vi "UDP Named Service - PS Server.vi"() -> ()   [LabVIEW 2025]
doc: "Creates a named service and listens on the first available port. When a client connects to the service, it sends a response string to the client.\nAuthor: Scott Hannahs <sth@magnet.fsu.edu>\n\nThis software is licensed for use under the “MIT License\"\nCopyright (c) 2025 Scott Hannahs, sth@sth@magnet.sthnet.net\n\nPermission is hereby granted, free of charge, to any person obtaining a copy of this software and associated documentation files (the \"Software\"), to deal in the Software without restriction, including without limitation the rights to use, copy, modify, merge, publish, distribute, sublicense, and/or sell copies of the Software, and to permit persons to whom the Software is furnished to do so, subject to the following conditions: The above copyright notice and this permission notice shall be included in all copies or substantial portions of the Software.\n\nTHE SOFTWARE IS PROVIDED \"AS IS\", WITHOUT WARRANTY OF ANY KIND, EXPRESS OR IMPLIED, INCLUDING BUT NOT LIMITED TO THE WARRANTIES OF MERCHANTABILITY, FITNESS FOR A PARTICULAR PURPOSE AND NONINFRINGEMENT. IN NO EVENT SHALL THE AUTHORS OR COPYRIGHT HOLDERS BE LIABLE FOR ANY CLAIM, DAMAGES OR OTHER LIABILITY, WHETHER IN AN ACTION OF CONTRACT, TORT OR OTHERWISE, ARISING FROM, OUT OF OR IN CONNECTION WITH THE SOFTWARE OR THE USE OR OTHER DEALINGS IN THE SOFTWARE."
uses:
  <vilib>/Utility/error.llb/Trim Whitespace One-Sided.vi
panel:
  out "Port":u16
  out "String":string
  in  "Stop":bool
  # "Overview: Demonstrates the use of the UDP functions to initialize a named UDP service that can send data to a client VI.\nInstructions:\n1. Run the VI.\n2. Open UDP Named Service - Client.vi and follow the instructions on its front panel.\n3. Click Stop to stop the VI."
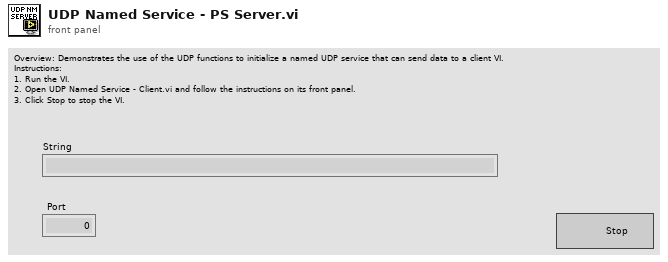
[diagram p1: front panel]
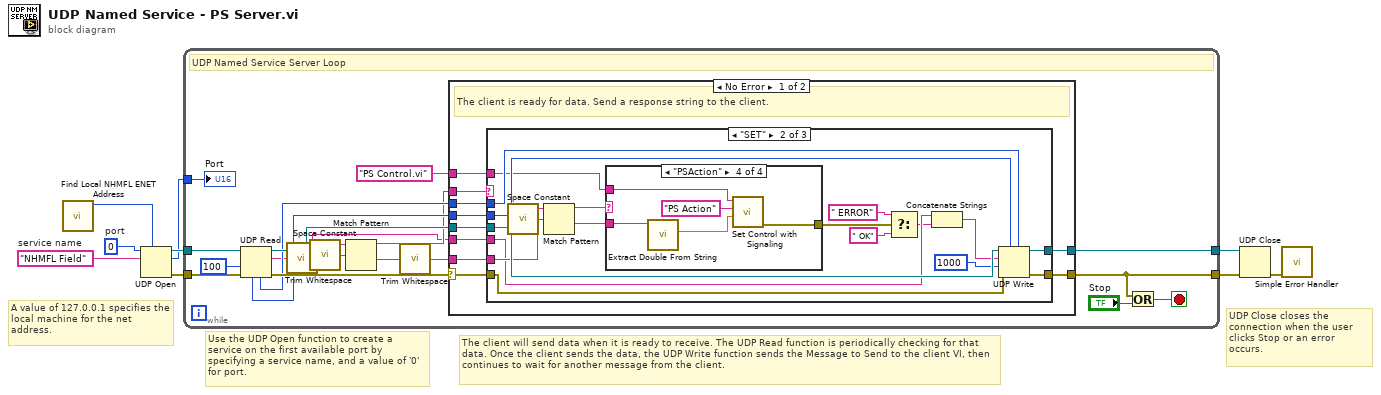
[diagram p0: block diagram]
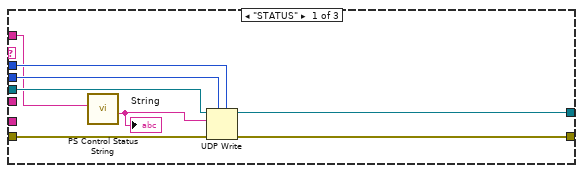
[diagram p2: hidden frame]
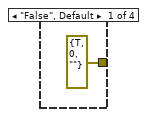
[diagram p3: hidden frame]
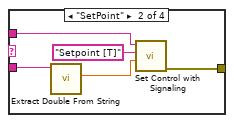
[diagram p4: hidden frame]
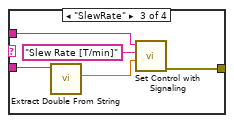
[diagram p5: hidden frame]
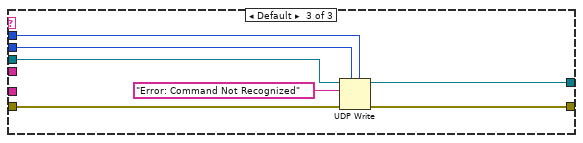
[diagram p6: hidden frame]
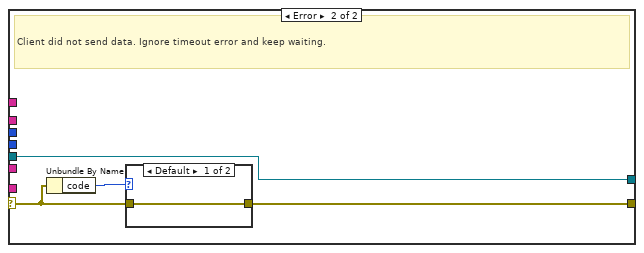
[diagram p7: hidden frame]
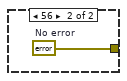
[diagram p8: hidden frame]
diagram:
  w2 = u16 0  # port
  w9 = "NHMFL Field"  # service name
  # "UDP Close closes the connection when the user clicks Stop or an error occurs."
  # "A value of 127.0.0.1 specifies the local machine for the net address."
  # "The client will send data when it is ready to receive. The UDP Read function is periodically checking for that data. Once the client sends the data, the UDP Write function sends the Message to Send to the client VI, then continues to wait for another message from the client."
  # "Use the UDP Open function to create a service on the first available port by specifying a service name, and a value of '0' for port."
  n1 = call "Find Local NHMFL ENET Address.vi"() -> ("Ethernet Address"=w1:u32)  [unwired: 9 in, 2 out]
  n2 = UDP Open(7:w1, 10:w9, 11:w2) -> (port=w8:refnum<k16>, 0:w7:errorcluster, 2:w4:u16)  [unwired: 2 in]
  n3 = while {
    tunnel: [w19] -> w5
    tunnel: w8 -> [w28]
    tunnel: w7 -> [w24]
    tunnel: [w25] -> w6
    tunnel: w4 -> [w22]
    stop <- w21 stop-if-true
    # "UDP Named Service Server Loop"
    n4 = UDP Read(connection ID=w28, timeout ms (25000)=100, 8:w24) -> (data out=w12:string, error out=w27:errorcluster, 3:w26:refnum<k16>, 4:w23:u16, 6:w17:u32)  [unwired: 1 in]
    n5 = call <vilib>:"Trim Whitespace.vi"("string"=w12) -> ("trimmed string"=w10:string)  [unwired: 1 in]
    n6 = call <vilib>:"Space Constant.vi"() -> ("String"=w13:string)
    n7 = Match Pattern(string=w10, regular expression=w13) -> (before substring=w16:string, after substring=w15:string)  [unwired: 1 in, 2 out]
    n8 = call <vilib>:"Trim Whitespace.vi"("string"=w15) -> ("trimmed string"=w14:string)  [unwired: 1 in]
    n9 = case shown="No Error" w27 {
      selector: w27 -> [w38 w90]
      tunnel: w26 -> [w35 w91]
      tunnel: [w37 w88] -> w19
      tunnel: [w36 w91] -> w25
      tunnel: w17 -> [w33 _]
      tunnel: w23 -> [w34 _]
      tunnel: w16 -> [w32 _]
      tunnel: w14 -> [w31 _]
      tunnel: w10 -> [w30 _]
      tunnel: "PS Control.vi" -> [w29 _]
      frame No Error {
        # "The client is ready for data. Send a response string to the client."
        n10 = case shown="\"SET\"" w32 {
          tunnel: w38 -> [w46 w64 w87]
          tunnel: [w45 w63 w86] -> w37
          tunnel: [w44 w62 w85] -> w36
          tunnel: w35 -> [w43 w61 w84]
          tunnel: w34 -> [w42 w60 w83]
          tunnel: w33 -> [w41 w59 w82]
          tunnel: w31 -> [_ w58 _]
          tunnel: w30 -> [_ w54 _]
          tunnel: w29 -> [w39 w47 _]
          frame "STATUS" {
            n11 = call "PS Control Status String.vi"("VI Name"=w39) -> ("Status String"=w40:string)  [unwired: 9 in, 1 out]
            "String" <- w40
            n12 = UDP Write(address=w41, port or service name=w42, connection ID=w43, data in=w40, 8:w46) -> (error out=w45:errorcluster, 3:w44:refnum<k16>)  [unwired: 1 in]
          }
          frame "SET" {
            n13 = call <vilib>:"Space Constant.vi"() -> ("String"=w57:string)
            n14 = Match Pattern(string=w58, regular expression=w57) -> (before substring=w56:string, after substring=w55:string)  [unwired: 1 in, 2 out]
            n15 = case shown="\"PSAction\"" w56 {
              tunnel: w55 -> [_ w67 w72 w77]
              tunnel: w47 -> [_ w69 w74 w79]
              tunnel: [errorcluster {"status"=TRUE, "code"=0, "source"=""} ("error out") w66 w71 w76] -> w53
              frame "False", Default {
              }
              frame "SetPoint" {
                n16 = call "Extract Double From String.vi"("string"=w67) -> ("floating pt. number"=w68:dbl)  [unwired: 3 in, 3 out]
                n17 = call "Set Control with Signaling.vi"("Value"=w68, "Control Name"="Setpoint [T]", "VI Name"=w69) -> ("error out"=w66:errorcluster)  [unwired: 8 in]
              }
              frame "SlewRate" {
                n18 = call "Extract Double From String.vi"("string"=w72) -> ("floating pt. number"=w73:dbl)  [unwired: 3 in, 3 out]
                n19 = call "Set Control with Signaling.vi"("Value"=w73, "Control Name"="Slew Rate [T/min]", "VI Name"=w74) -> ("error out"=w71:errorcluster)  [unwired: 8 in]
              }
              frame "PSAction" {
                n20 = call "Extract Double From String.vi"("string"=w77) -> ("floating pt. number"=w78:dbl)  [unwired: 3 in, 3 out]
                n21 = call "Set Control with Signaling.vi"("Value"=w78, "Control Name"="PS Action", "VI Name"=w79) -> ("error out"=w76:errorcluster)  [unwired: 8 in]
              }
            }
            n22 = Select(t=" ERROR", s=w53, f=" OK") -> (s? t:f=w49:string)
            n23 = Concatenate Strings(w54, w49) -> (w48:string)
            n24 = UDP Write(address=w59, port or service name=w60, connection ID=w61, data in=w48, 8:w64, 9:1000 ("timeout ms (25000)")) -> (error out=w63:errorcluster, 3:w62:refnum<k16>)
          }
          frame Default {
            n25 = UDP Write(address=w82, port or service name=w83, connection ID=w84, data in="Error: Command Not Recognized", 8:w87) -> (error out=w86:errorcluster, 3:w85:refnum<k16>)  [unwired: 1 in]
          }
        }
      }
      frame Error {
        # "Client did not send data. Ignore timeout error and keep waiting."
        n26 = Unbundle By Name(w90) -> ("code"=w89:i32)
        n27 = case shown="Default" w89 {
          tunnel: w90 -> [w92 _]
          tunnel: [w92 w93] -> w88
          frame Default {
          }
          frame 56 {
            w93 = errorcluster {"status"=FALSE, "code"=0, "source"=""}  # No error
          }
        }
      }
    }
    n28 = Or(x=w19, y="Stop") -> (x .or. y?=w21:bool)
    "Port" <- w22
  }
  n29 = UDP Close(connection ID=w6, 8:w5) -> (error out=w3:errorcluster)  [unwired: 1 out]
  n30 = call <vilib>:"Simple Error Handler.vi"("error in (no error)"=w3) -> ()  [unwired: 4 in, 5 out]
